vi "Get Option String.vi"(0 "FPGA File Path":path, 5 "Suppress System Calibration?":bool) -> (4 "RFmx Option String":string, 6 "FPGA Option String":string, 8 "RFPM Option String":string)   [LabVIEW 2023, in "RFFixtureCharact.RFPM.lvlib" / "RF Subsystem Session Provider.lvclass"]
uses:
  RF Subsystem Session Provider.lvclass
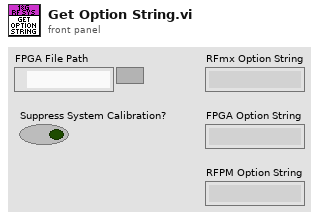
[diagram p1: front panel]
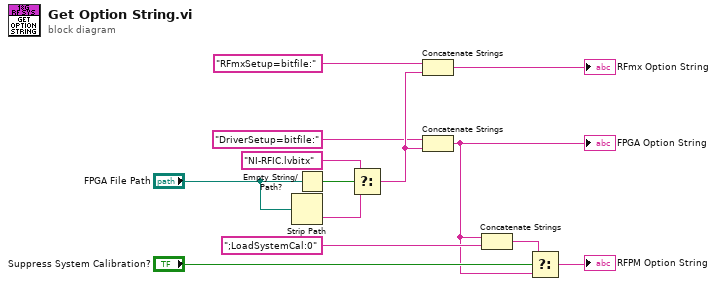
[diagram p0: block diagram]
diagram:
  n1 = Strip Path(path="FPGA File Path") -> (name=w6:string)  [unwired: 1 out]
  n2 = Empty String/Path?(string/path="FPGA File Path") -> (empty?=w8:bool)
  n3 = Select(t="NI-RFIC.lvbitx", s=w8, f=w6) -> (s? t:f=w9:string)
  n4 = Concatenate Strings("RFmxSetup=bitfile:", w9) -> (→"RFmx Option String":string)
  n5 = Concatenate Strings("DriverSetup=bitfile:", w9) -> (w1:string)
  "FPGA Option String" <- w1
  n6 = Concatenate Strings(w1, ";LoadSystemCal:0") -> (w12:string)
  n7 = Select(t=w12, s="Suppress System Calibration?", f=w1) -> (s? t:f=→"RFPM Option String":string)
